vi "test_output_dual_pid.vi"() -> ()   [LabVIEW 2013]
panel:
  out "size(s)":i32[](array[numeric])
  out "Waveform Graph 2":i16[](graph)
  out "Waveform Graph":dbl[][](graph)
  in  "Output mixer fequency [MHz]":dbl
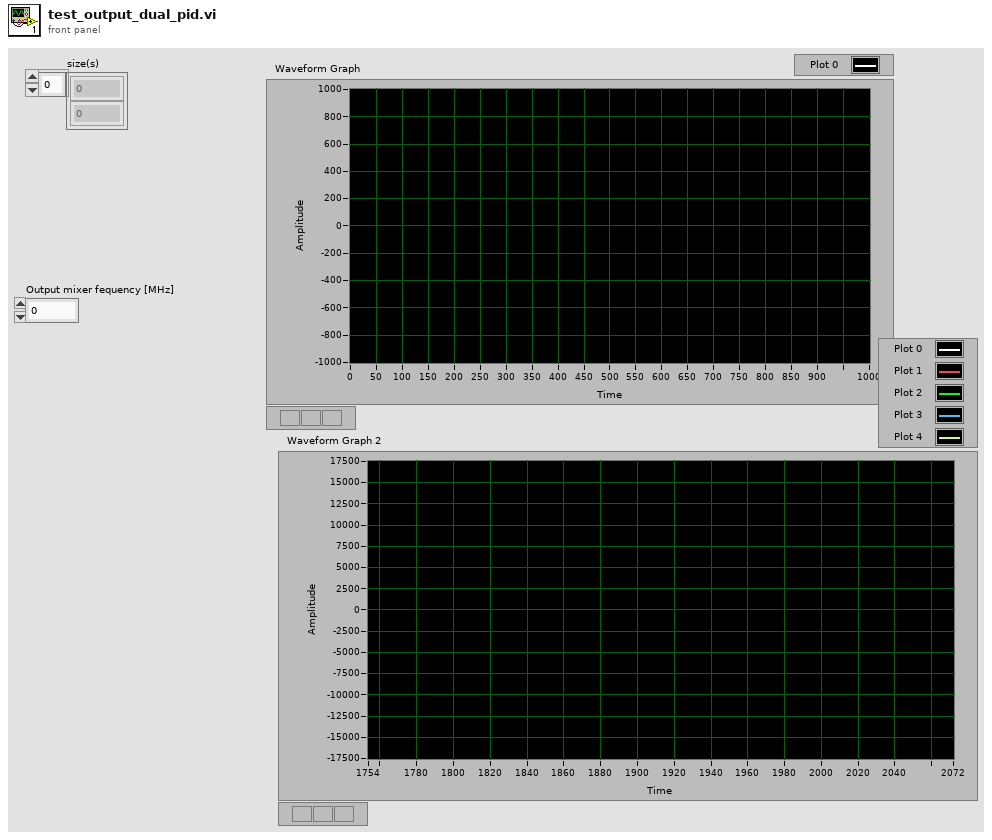
[diagram p1: front panel]
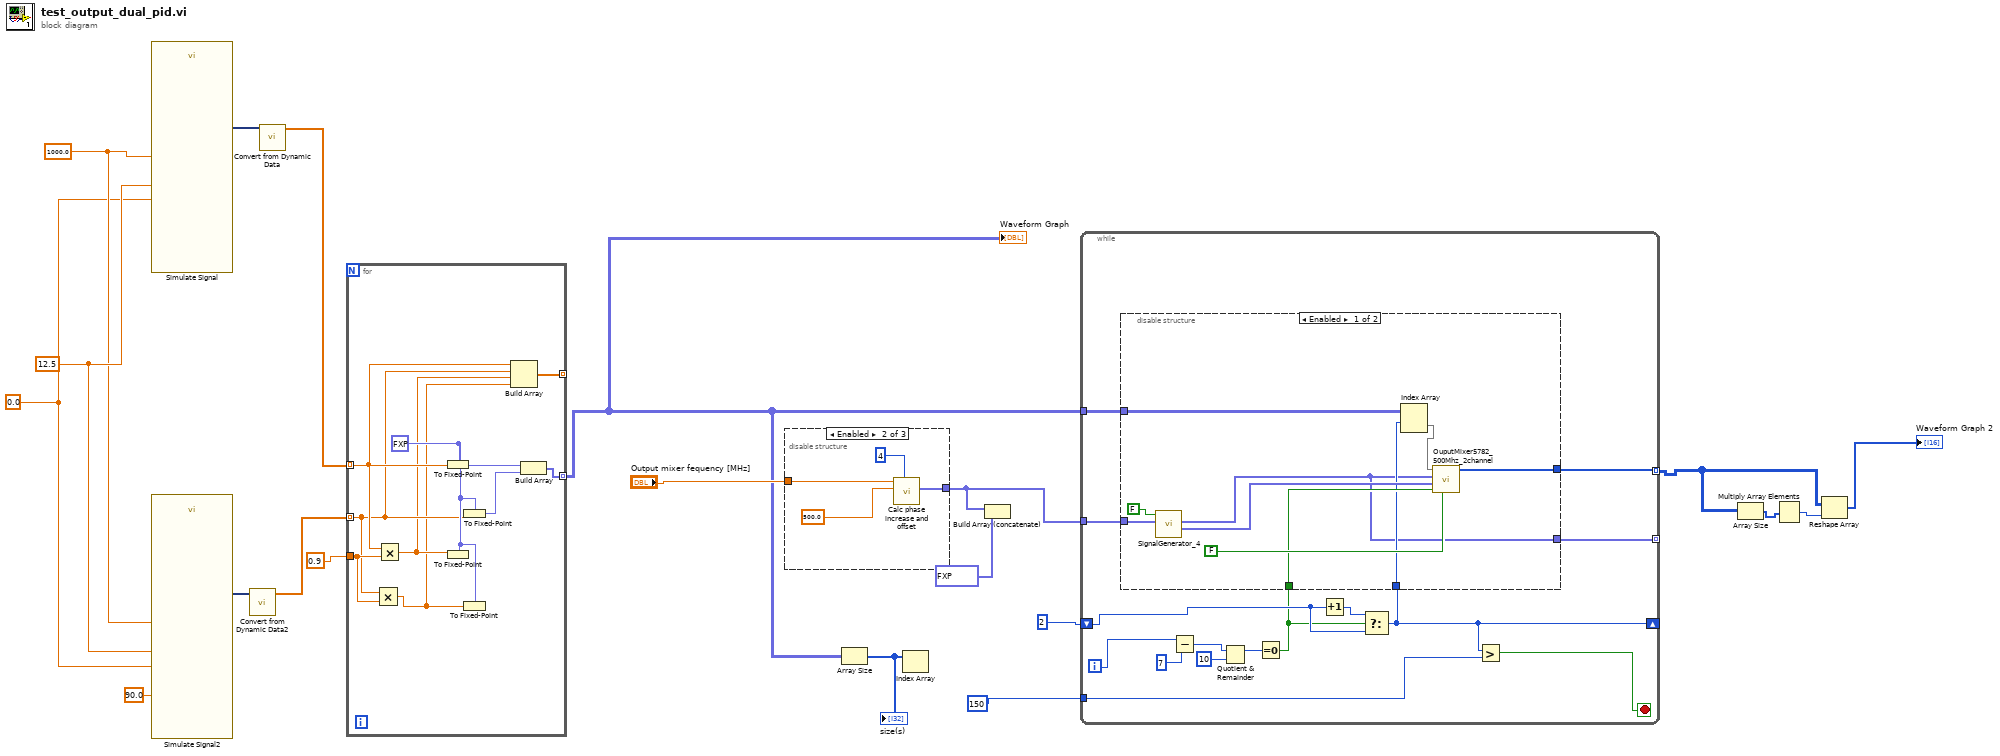
[diagram p0: block diagram]
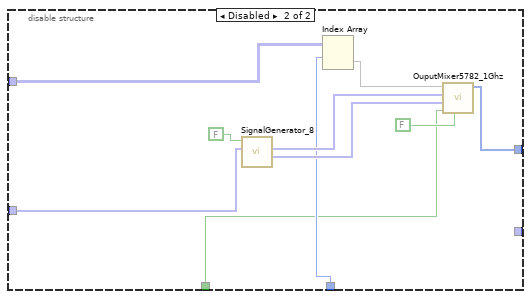
[diagram p2: hidden frame]
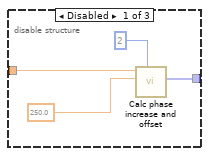
[diagram p3: hidden frame]
diagram:
  w12 = 1000.0 ("Amplitude")
  w13 = 12.5 ("Frequency")
  w10 = 0.0 ("Noise amplitude")
  n1 = call "Simulate Signal"("Frequency"=w13, "Amplitude"=w12, "Noise amplitude"=w10) -> ("Sine with Uniform Noise"=w18:dynamicdata)  [unwired: 11 in, 1 out]
  n2 = call "Simulate Signal2"("Frequency"=w13, "Amplitude"=w12, "Phase"=90.0, "Noise amplitude"=w10) -> ("Sine with Uniform Noise"=w16:dynamicdata)  [unwired: 10 in, 1 out]
  n3 = call "Convert from Dynamic Data2"("Dynamic Data Type"=w16) -> ("Array"=w14:dbl[])  [unwired: 3 in]
  n4 = call "Convert from Dynamic Data"("Dynamic Data Type"=w18) -> ("Array"=w15:dbl[])  [unwired: 3 in]
  n5 = for {
    tunnel: w14 -> [w24] mode=indexing
    tunnel: w15 -> [w25] mode=indexing
    tunnel: [w28] -> w7 mode=indexing
    tunnel: 0.9 ("y") -> [w27]
    tunnel: [w21] -> _ mode=indexing
    w26 = fxp<+/-,16,14> 0.0 ("f")
    n6 = Multiply(x=w24, y=w27) -> (x*y=w22:dbl)
    n7 = Multiply(x=w25, y=w27) -> (x*y=w23:dbl)
    n8 = To Fixed-Point(fixed-point type=w26, number=w25) -> (fixed-point=w30:fxp<+/-,16,14>)
    n9 = To Fixed-Point(fixed-point type=w26, number=w23) -> ()  [unwired: 1 out]
    n10 = To Fixed-Point(fixed-point type=w26, number=w24) -> (fixed-point=w29:fxp<+/-,16,14>)
    n11 = To Fixed-Point(fixed-point type=w26, number=w22) -> ()  [unwired: 1 out]
    n12 = Build Array(w25, w24, w23, w22) -> (w21:dbl[])
    n13 = Build Array(w30, w29) -> (w28:fxp<+/-,16,14>[])
  }
  "Waveform Graph" <- w7
  n14 = disable-structure shown="Enabled" {
    disable-tunnel: [w32 w36 _] -> w1
    disable-tunnel: "Output mixer fequency [MHz]" -> [w31 w35 _]
    frame Disabled {
      n15 = call "Calc phase increase and offset.vi"("# of DDS"=2, "fclk (MHz)"=250.0 ("fclk (800MHz)"), "f_generated (MHz)"=w31) -> ("Phase out"=w32:fxp<+,64,64>[])  [unwired: 6 in, 2 out]
    }
    frame Enabled {
      n16 = call "Calc phase increase and offset.vi"("# of DDS"=4, "fclk (MHz)"=500.0 ("fclk (800MHz)"), "f_generated (MHz)"=w35) -> ("Phase out"=w36:fxp<+,64,64>[])  [unwired: 6 in, 2 out]
    }
    frame Disabled {
    }
  }
  n17 = Array Size(array=w7) -> (size(s)=w8:i32[])
  "size(s)" <- w8
  n18 = Index Array(array=w8) -> ()  [unwired: 1 in, 1 out]
  n19 = Build Array (concatenate)(w1, fxp<+,64,64>[] [0.0, 0.0, 0.0, 0.0] ("array")) -> ()  [unwired: 1 out]
  n20 = while {
    tunnel: w1 -> [w53]
    tunnel: w7 -> [w45]
    shift-right: [w40] -> _
    shift-left: 2 ("y") -> [w47]
    tunnel: [w43] -> w3 mode=indexing
    tunnel: 150 -> [w42]
    tunnel: [w39] -> _ mode=indexing
    i -> [w44]
    stop <- w41 stop-if-true
    n21 = Subtract(x=w44, y=7) -> (x-y=w48:i32)
    n22 = Quotient & Remainder(x=w48, y=10) -> (x-y*floor(x/y)=w51:i32)  [unwired: 1 out]
    n23 = Equal To 0?(x=w51) -> (x = 0?=w46:bool)
    n24 = Increment(x=w47) -> (x+1=w50:i32)
    n25 = Select(t=w50, s=w46, f=w47) -> (s? t:f=w40:i32)
    n26 = disable-structure shown="Enabled" {
      disable-tunnel: w53 -> [w60 w65]
      disable-tunnel: w46 -> [w59 w64]
      disable-tunnel: w45 -> [w58 w69]
      disable-tunnel: [w56 w66] -> w43
      disable-tunnel: w40 -> [w55 w68]
      disable-tunnel: [w54 _] -> w39
      frame Enabled {
        n27 = call "SignalGenerator_4.vi"("Phase"=w60, "reset"=FALSE) -> ("Sine out"=w61:fxp<+/-,16,0>[], "Cosine out"=w54:fxp<+/-,16,0>[])  [unwired: 8 in]
        n28 = Index Array(array=w58, index (row)=w55) -> (element=w57:fxp<+/-,16,14>[])  [unwired: 1 in]
        n29 = call "OuputMixer5782_500Mhz_2channel.vi"("reset"=FALSE, "valid in"=w59, "Sine in"=w61, "Cosine in"=w54, "Data in"=w57) -> ("appended array"=w56:i16[])  [unwired: 5 in, 1 out]
      }
      frame Disabled {
        n30 = call "SignalGenerator_8.vi"("Phase"=w65, "reset"=FALSE) -> ("Sine out"=w70:fxp<+/-,16,0>[], "Cosine out"=w71:fxp<+/-,16,0>[])  [unwired: 8 in]
        n31 = Index Array(array=w69, index (row)=w68) -> (element=w67:fxp<+/-,16,14>[])  [unwired: 1 in]
        n32 = call "OuputMixer5782_1Ghz.vi"("reset"=FALSE, "valid in"=w64, "Sine in"=w70, "Cosine in"=w71, "Data in"=w67) -> ("test"=w66:i16[])  [unwired: 5 in, 1 out]
      }
    }
    n33 = Greater?(x=w40, y=w42) -> (0:w41:bool)
  }
  n34 = Array Size(array=w3) -> (size(s)=w5:i32[])
  n35 = Multiply Array Elements(1:w5) -> (0:w4:i32)
  n36 = Reshape Array(w3, w4) -> (→"Waveform Graph 2":i16[])
